vi "Write Pitch Data.vi"(11 "Pitch Calib":T1={"Array"=[[80.0, 0.9, 1.0, 1.0, 1.0, 1.0, 1.0, 1.0, 1.0], [70.0, 0.96, 0.0, 0.0, 0.0, 0.0, 0.0, 0.0, 0.0], [60.0, 1.08, 0.0, 0.0, 0.0, 0.0, 0.0, 0.0, 0.0], [50.0, 1.25, 0.0, 0.0, 0.0, 0.0, 0.0, 0.0, 0.0], [40.0, 1.44, 0.0, 0.0, 0.0, 0.0, 0.0, 0.0, 0.0], [30.0, 1.68, 0.0, 0.0, 0.0, 0.0, 0.0, 0.0, 0.0], [20.0, 1.91, 0.0, 0.0, 0.0, 0.0, 0.0, 0.0, 0.0], [10.0, 2.19, 0.0, 0.0, 0.0, 0.0, 0.0, 0.0, 0.0], [0.0, 2.47, 0.0, 0.0, 0.0, 0.0, 0.0, 0.0, 0.0], [-10.0, 2.73, 0.0, 0.0, 0.0, 0.0, 0.0, 0.0, 0.0], [-20.0, 3.01, 0.0, 0.0, 0.0, 0.0, 0.0, 0.0, 0.0], [-30.0, 3.3, 0.0, 0.0, 0.0, 0.0, 0.0, 0.0, 0.0], [-40.0, 3.5, 0.0, 0.0, 0.0, 0.0, 0.0, 0.0, 0.0], [-50.0, 3.72, 0.0, 0.0, 0.0, 0.0, 0.0, 0.0, 0.0], [-60.0, 3.92, 0.0, 0.0, 0.0, 0.0, 0.0, 0.0, 0.0], [-70.0, 4.05, 0.0, 0.0, 0.0, 0.0, 0.0, 0.0, 0.0], [-80.0, 4.11, 0.0, 0.0, 0.0, 0.0, 0.0, 0.0, 0.0]], "Operation"=FALSE}) -> ()   [LabVIEW 2017]
uses:
  Pitch Array 1.ctl
  <vilib>/Utility/file.llb/Write Delimited Spreadsheet (DBL).vi
panel:
  # "Calibration\nMode"
  # "Operating\nMode"
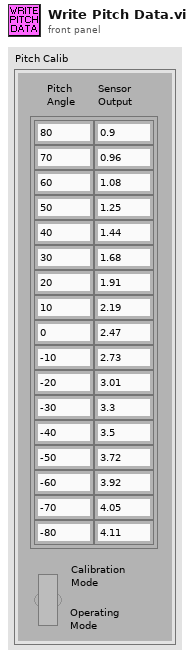
[diagram p1: front panel]
types:
  T1 = typedef "Pitch Array 1.ctl" = cluster{"Array":dbl[][], "Operation":bool}
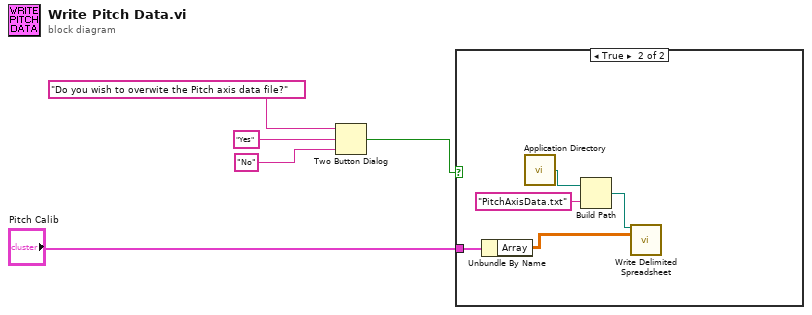
[diagram p0: block diagram]
diagram:
  n1 = Two Button Dialog(message="Do you wish to overwite the Pitch axis data file?", 1:"No" ("F button name (\"Cancel\")"), 2:"Yes" ("T button name (\"OK\")")) -> (T button?=w2:bool)
  n2 = case shown="True" w2 {
    tunnel: "Pitch Calib" -> [_ w10]
    frame False {
    }
    frame True {
      n3 = Unbundle By Name(w10) -> ("Array"=w9:dbl[][])
      n4 = call <vilib>:"Application Directory.vi"() -> ("Application Directory"=w8:path)
      n5 = Build Path(base path=w8, name or relative path="PitchAxisData.txt") -> (appended path=w7:path)
      n6 = call-poly <vilib>:"Write Delimited Spreadsheet.vi"("file path (dialog if empty)"=w7, "2D data"=w9) -> ()  [unwired: 12 in, 2 out]
    }
  }
